vi "Valid Measurement Service Name.vi"(8 "error in":errorcluster, 10 "Requested Plugin Name":string, 11 "Project ref":refnum<vi>) -> (0 "error out":errorcluster, 3 "Valid Name?":bool)   [LabVIEW 2020, in "MeasurementService Editor.lvlib"]
uses:
  MeasurementService Editor.lvlib
  48953c88-0603-4c13-ba6a-df914321b09e.vi
  <vilib>/Comparison/Equal/Equal Functor/Equal Functor.lvclass
panel:
  out "control chars":string
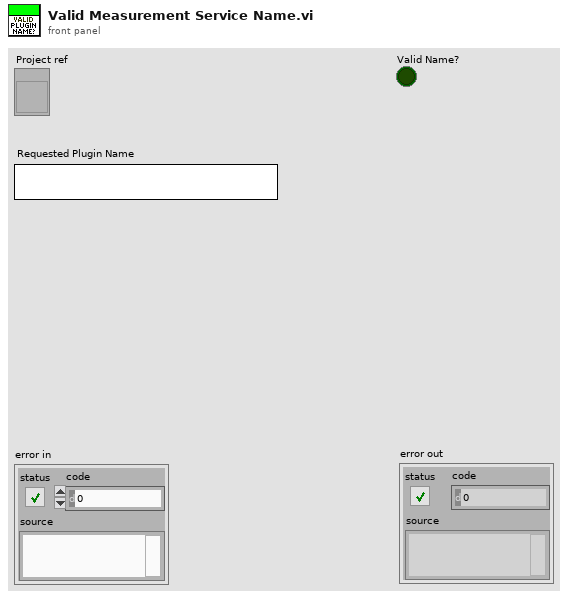
[diagram p1: front panel]
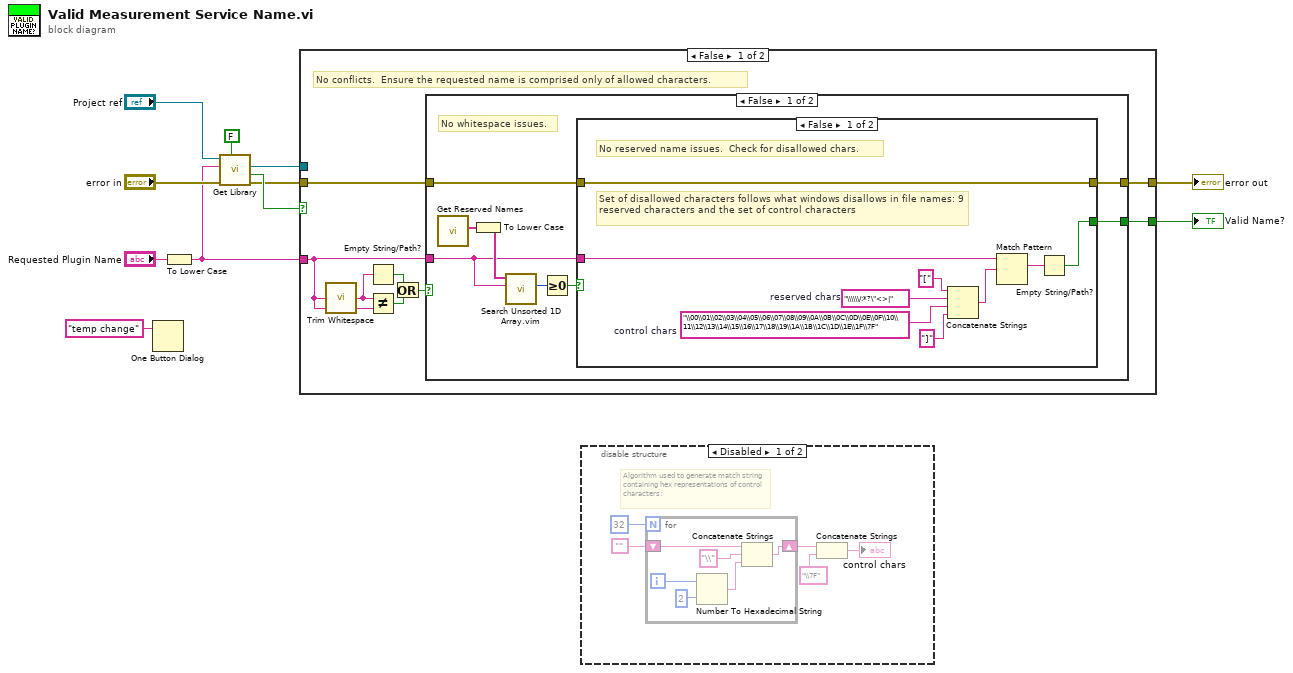
[diagram p0: block diagram]
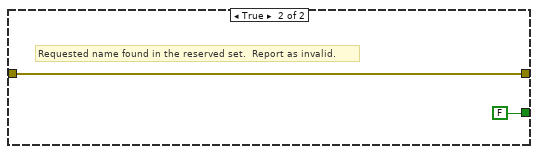
[diagram p3: hidden frame]
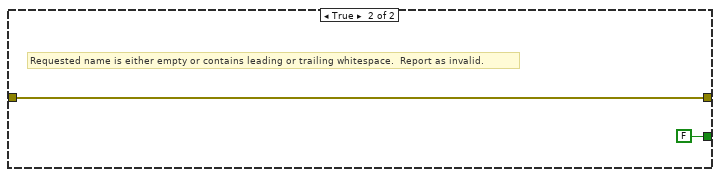
[diagram p4: hidden frame]
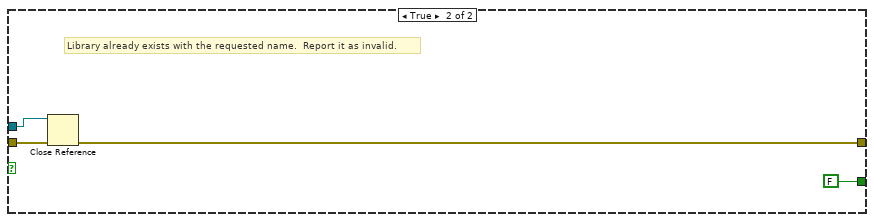
[diagram p5: hidden frame]
diagram:
  n1 = One Button Dialog(message="temp change") -> ()  [unwired: 1 in, 1 out]
  n2 = To Lower Case(string="Requested Plugin Name") -> (all lower case string=w2:string)
  n3 = call "Get Library.vi"("Error if not Found (T)"=FALSE, "error in (no error)"="error in", "Library Name"=w2, "Project in"="Project ref") -> ("error out"=w8:errorcluster, "Found"=w9:bool, "Library Item"=w7:refnum<vi>)  [unwired: 5 in]
  n4 = case shown="False" w9 {
    tunnel: w8 -> [w19 w44]
    tunnel: w7 -> [_ w42]
    tunnel: [w18 w43] -> w5
    tunnel: [w17 FALSE ("Valid Name?")] -> w4
    tunnel: w2 -> [w12 _]
    frame False {
      # "No conflicts.  Ensure the requested name is comprised only of allowed characters."
      n5 = call <vilib>:"Trim Whitespace.vi"("string"=w12) -> ("trimmed string"=w16:string)  [unwired: 1 in]
      n6 = Empty String/Path?(string/path=w16) -> (empty?=w14:bool)
      n7 = Not Equal?(x=w16, y=w12) -> (x != y?=w15:bool)
      n8 = Or(x=w14, y=w15) -> (x .or. y?=w13:bool)
      n9 = case shown="False" w13 {
        tunnel: w12 -> [w23 _]
        tunnel: w19 -> [w27 w40]
        tunnel: [w26 w40] -> w18
        tunnel: [w20 FALSE ("Error if not Found (T)")] -> w17
        frame False {
          # "No whitespace issues."
          n10 = call "Get Reserved Names.vi"() -> ("Reserved names"=w25:string[])  [unwired: 11 in]
          n11 = To Lower Case(string=w25) -> (all lower case string=w24:string[])
          n12 = call "Search Unsorted 1D Array.vim"("element"=w23, "unsorted 1D array"=w24) -> ("index of element"=w22:i32)  [unwired: 9 in]
          n13 = Greater Or Equal To 0?(x=w22) -> (x >= 0?=w21:bool)
          n14 = case shown="False" w21 {
            tunnel: w23 -> [w35 _]
            tunnel: w27 -> [w36 w38]
            tunnel: [w36 w38] -> w26
            tunnel: [w33 FALSE ("Error if not Found (T)")] -> w20
            frame False {
              w28 = "\\00\\01\\02\\03\\04\\05\\06\\07\\08\\09\\0A\\0B\\0C\\0D\\0E\\0F\\10\\11\\12\\13\\14\\15\\16\\17\\18\\19\\1A\\1B\\1C\\1D\\1E\\1F\\7F"  # control chars
              w32 = "\\\\\\/:*?\"<>|"  # reserved chars
              # "Set of disallowed characters follows what windows disallows in file names: 9 reserved characters and the set of control characters"
              # "No reserved name issues.  Check for disallowed chars."
              n15 = Concatenate Strings("[" ("string"), w32, w28, "]" ("string")) -> (w29:string)
              n16 = Match Pattern(string=w35, regular expression=w29) -> (match substring=w34:string)  [unwired: 1 in, 3 out]
              n17 = Empty String/Path?(string/path=w34) -> (empty?=w33:bool)
            }
            frame True {
              # "Requested name found in the reserved set.  Report as invalid."
            }
          }
        }
        frame True {
          # "Requested name is either empty or contains leading or trailing whitespace.  Report as invalid."
        }
      }
    }
    frame True {
      # "Library already exists with the requested name.  Report it as invalid."
      n18 = Close Reference(reference=w42, error in (no error)=w44) -> (error out=w43:errorcluster)
    }
  }
  "error out" <- w5
  "Valid Name?" <- w4
  n19 = disable-structure shown="Disabled" {
    frame Disabled {
      # "Algorithm used to generate match string containing hex representations of control characters:"
      n20 = for {
        N: 32 -> [_]
        shift-right: [w51] -> w47
        shift-left: "" -> [w50]
        i -> [w55]
        n21 = Number To Hexadecimal String(1:i16 2 ("width (-)"), 2:w55) -> (0:w53:string)
        n22 = Concatenate Strings(w50, "\\" ("string"), w53) -> (w51:string)
      }
      n23 = Concatenate Strings(w47, "\\7F") -> (→"control chars":string)
    }
    frame Enabled {
    }
  }
